vi "Open SystemLink Tag.vi"(6 "Connection Type":T2, 8 "error in (no error)":errorcluster, 9 "Path":string, 10 "Data Tag Type":T1, 11 "NI Skyline Configuration in":refnum<class "NI Skyline Configuration.lvclass">) -> (0 "error out":errorcluster, 3 "NI Skyline Tag out":refnum<class "NI Skyline Tag.lvclass">)   [LabVIEW 2015, in "SystemLink File runtime.lvclass"]
doc: "Open SystemLink Tag Connection"
uses:
  SystemLink File runtime.lvclass
  configuration/Connection Type.ctl
  <vilib>/Skyline/Configuration/Configuration_class/NI Skyline Configuration.lvclass
  configuration/Data Tag Type.ctl
  <vilib>/Skyline/Tag/Wrapper/Wrapper_class/NI Skyline Tag.lvclass
  <vilib>/Skyline/Configuration/Configuration HTTP_class/NI Skyline Configuration HTTP.lvclass
  <vilib>/Skyline/Configuration/Configuration AMQP_class/NI Skyline Configuration AMQP.lvclass
  <vilib>/Skyline/Tag/Wrapper/Wrapper HTTP_class/Open Tag HTTP.vi
  <vilib>/Skyline/Tag/Wrapper/Wrapper AMQP_class/Open Tag AMQP.vi
  configuration/SystemLink File configuration.lvclass
  <vilib>/Skyline/Tag/Wrapper/Wrapper AMQP_class/NI Skyline Tag AMQP.lvclass
  <vilib>/Skyline/Tag/Wrapper/Wrapper HTTP_class/NI Skyline Tag HTTP.lvclass
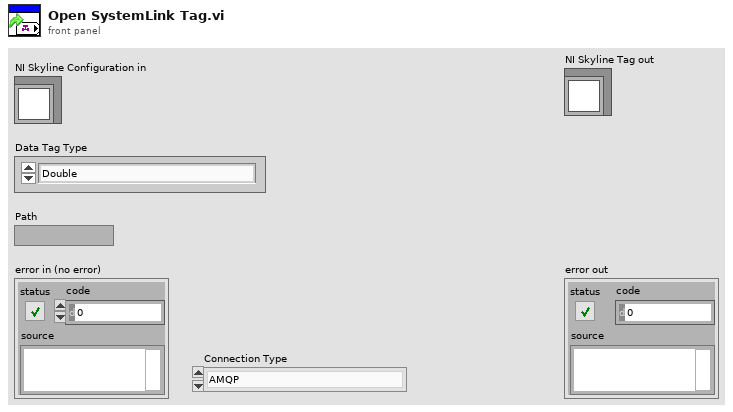
[diagram p1: front panel]
types:
  T1 = typedef "SystemLink File configuration.lvclass/Data Tag Type.ctl" = enum16{"Double", "Single", "I32", "I16", "I8", "U64", "U32", "U16", "U8", "Boolean", "String", "Timestamp"}
  T2 = typedef "SystemLink File configuration.lvclass/Connection Type.ctl" = enum16{"AMQP", "HTTP", "API Key (SystemLink Cloud)"}
  T3 = typedef "NI Skyline Tag.lvlib/DataType.ctl" = enum32{"Double", "I32", "String", "Boolean", "U64", "Timestamp"}
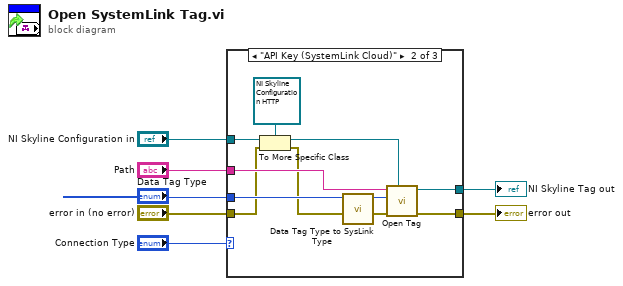
[diagram p0: block diagram]
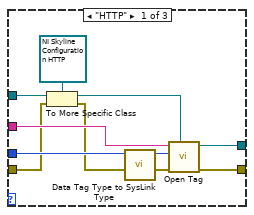
[diagram p2: hidden frame]
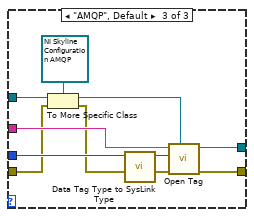
[diagram p3: hidden frame]
diagram:
  n1 = case shown="\"API Key (SystemLink Cloud)\"" "Connection Type" {
    tunnel: "NI Skyline Configuration in" -> [w17 w27 w37]
    tunnel: "Data Tag Type" -> [w16 w26 w36]
    tunnel: "Path" -> [w15 w25 w35]
    tunnel: [w14 w24 w34] -> w4
    tunnel: "error in (no error)" -> [w10 w20 w30]
    tunnel: [w13 w23 w33] -> w2
    frame "HTTP" {
      n2 = To More Specific Class(target class=refnum<class "NI Skyline Configuration HTTP.lvclass"> refnum ("configuration"), reference=w17, error in=w10) -> (specific class reference=w11:refnum<class "NI Skyline Configuration HTTP.lvclass">, error out=w9:errorcluster)
      n3 = call "Data Tag Type to SysLink Type.vi"("Data Tag Type"=w16) -> ("data type"=w12:T3)  [unwired: 10 in]
      n4 = call-poly <vilib>:"Open Tag.vi"("configuration"=w11, "error in (no error)"=w9, "Data Type"=w12, "path"=w15) -> ("error out"=w14:errorcluster, "tag out"=w13:refnum<class "NI Skyline Tag.lvclass">)  [unwired: 6 in]
    }
    frame "API Key (SystemLink Cloud)" {
      n5 = To More Specific Class(target class=refnum<class "NI Skyline Configuration HTTP.lvclass"> refnum ("configuration"), reference=w27, error in=w20) -> (specific class reference=w21:refnum<class "NI Skyline Configuration HTTP.lvclass">, error out=w19:errorcluster)
      n6 = call "Data Tag Type to SysLink Type.vi"("Data Tag Type"=w26) -> ("data type"=w22:T3)  [unwired: 10 in]
      n7 = call-poly <vilib>:"Open Tag.vi"("configuration"=w21, "error in (no error)"=w19, "Data Type"=w22, "path"=w25) -> ("error out"=w24:errorcluster, "tag out"=w23:refnum<class "NI Skyline Tag.lvclass">)  [unwired: 6 in]
    }
    frame "AMQP", Default {
      n8 = To More Specific Class(target class=refnum<class "NI Skyline Configuration AMQP.lvclass"> refnum ("configuration"), reference=w37, error in=w30) -> (specific class reference=w31:refnum<class "NI Skyline Configuration AMQP.lvclass">, error out=w29:errorcluster)
      n9 = call "Data Tag Type to SysLink Type.vi"("Data Tag Type"=w36) -> ("data type"=w32:T3)  [unwired: 10 in]
      n10 = call-poly <vilib>:"Open Tag.vi"("configuration"=w31, "error in (no error)"=w29, "data type"=w32, "path"=w35) -> ("error out"=w34:errorcluster, "tag out"=w33:refnum<class "NI Skyline Tag.lvclass">)  [unwired: 6 in]
    }
  }
  "error out" <- w4
  "NI Skyline Tag out" <- w2
